vi "findLocation.vi"(10 "DAQmx \nPhysical Channel":tag="Dev2/ai0:31") -> (1 "Animals location":string)   [LabVIEW 2017]
panel:
  out "x/y 2":dbl
  out "max value":dbl
  out "sum":dbl
  out "max\nweights":dbl[](array[numeric])
  out "voltsPerGram":dbl[](array[numeric])
  out "zeroSignals":dbl[](array[numeric])
  out "load cell\nsignal":dbl[](array[numeric])
  in  "number of consecutive\nmeasurements":i32=10
  out "array w/ subset deleted":dbl[][](array[numeric])
  out "min \nweights":dbl[](array[numeric])
  out "appended array":dbl[][](array[numeric])
  out "x/y":dbl[](array[numeric])
  # "should be 10 for the rats"
  # "Channels to weigh"
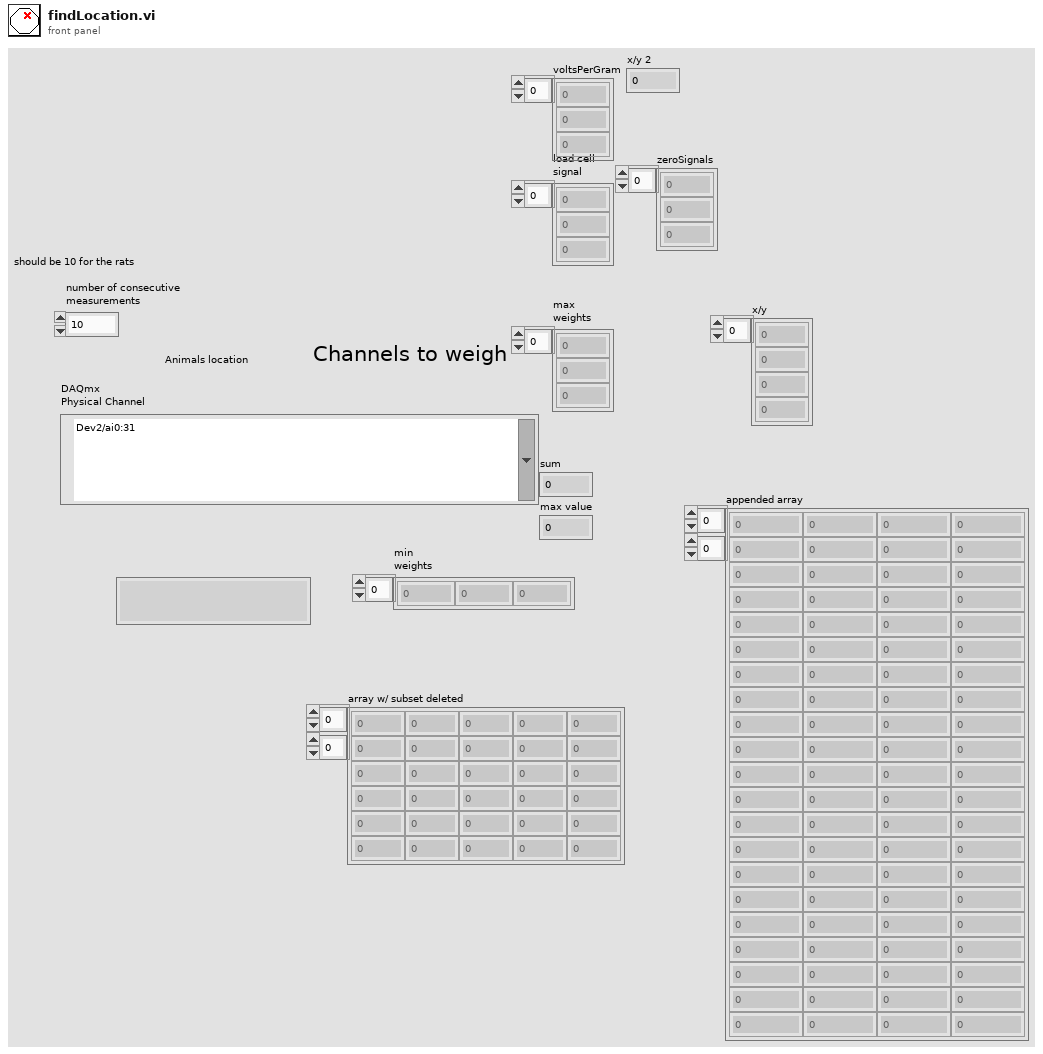
[diagram p1: front panel]
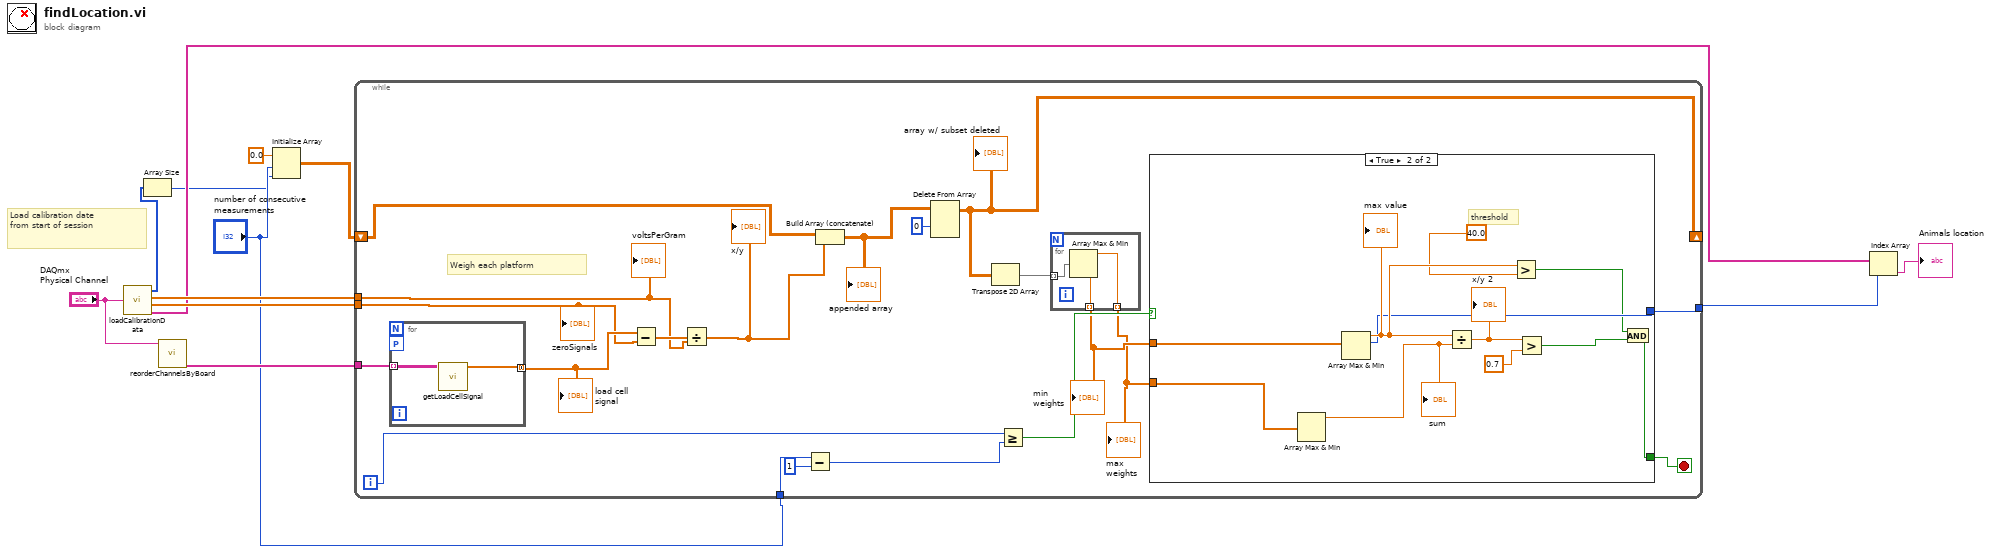
[diagram p0: block diagram]
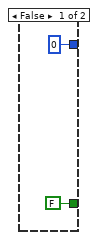
[diagram p2: hidden frame]
diagram:
  # "Load calibration date\nfrom start of session"
  n1 = call "loadCalibrationData.vi"("DAQmx \nPhysical Channel"="DAQmx \nPhysical Channel") -> ("channel names out"=w7:string[], "zeroSignals"=w12:dbl[], "voltsPerGram"=w11:dbl[], "index"=w4:i32[])  [unwired: 7 in]
  n2 = Array Size(array=w4) -> (size(s)=w1:i32)
  n3 = call "reorderChannelsByBoard.vi"("DAQmx \nPhysical Channel"="DAQmx \nPhysical Channel") -> ("Separated inputs\nas strings"=w9:string[])  [unwired: 8 in, 2 out]
  n4 = Initialize Array(0.0 ("element"), "number of consecutive\nmeasurements", w1) -> (w3:dbl[][])
  n5 = while {
    tunnel: w12 -> [w26]
    tunnel: w11 -> [w31]
    tunnel: w9 -> [w29]
    tunnel: [w28] -> w8
    shift-right: [w15] -> _
    shift-left: w3 -> [w24]
    tunnel: "number of consecutive\nmeasurements" -> [w17]
    i -> [w22]
    stop <- w27 stop-if-true
    # "Weigh each platform"
    n6 = for {
      workers-P: _ -> [_]
      tunnel: w29 -> [w50] mode=indexing
      tunnel: [w49] -> w30 mode=concatenating
      n7 = call "getLoadCellSignal.vi"("DAQmx Physical Channel"=w50) -> ("load cell\nsignal"=w49:dbl[])  [unwired: 10 in]
    }
    "load cell\nsignal" <- w30
    n8 = Subtract(x=w30, y=w26) -> (x-y=w32:dbl[])
    n9 = Divide(x=w32, y=w31) -> (x/y=w25:dbl[])
    "x/y" <- w25
    n10 = Subtract(x=w17, y=1) -> (x-y=w14:i32)
    n11 = Build Array (concatenate)(w24, w25) -> (w21:dbl[][])
    "appended array" <- w21
    n12 = Delete From Array(array=w21, index (row)=0) -> (array with subset deleted=w15:dbl[][])  [unwired: 2 in, 1 out]
    "array w/ subset deleted" <- w15
    n13 = Transpose 2D Array(2D array=w15) -> (transposed array=w18:dbl[][])
    n14 = Greater Or Equal?(x=w22, y=w14) -> (x >= y?=w23:bool)
    n15 = for {
      tunnel: w18 -> [w35] mode=indexing
      tunnel: [w34] -> w20 mode=indexing
      tunnel: [w33] -> w13 mode=indexing
      n16 = Array Max & Min(array=w35) -> (max value=w33:dbl, min value=w34:dbl)  [unwired: 2 out]
    }
    "min \nweights" <- w20
    "max\nweights" <- w13
    n17 = case shown="True" w23 {
      tunnel: [0 w42] -> w28
      tunnel: [FALSE w44] -> w27
      tunnel: w20 -> [_ w43]
      tunnel: w13 -> [_ w39]
      frame False {
      }
      frame True {
        # "threshold"
        n18 = Array Max & Min(array=w39) -> (max value=w38:dbl)  [unwired: 3 out]
        "sum" <- w38
        n19 = Array Max & Min(array=w43) -> (max value=w46:dbl, max index (indices)=w42:i32)  [unwired: 2 out]
        "max value" <- w46
        n20 = Divide(x=w46, y=w38) -> (x/y=w48:dbl)
        "x/y 2" <- w48
        n21 = Greater?(x=w46, y=40.0) -> (0:w40:bool)
        n22 = Greater?(x=w48, y=0.7) -> (0:w45:bool)
        n23 = And(x=w40, y=w45) -> (x .and. y?=w44:bool)
      }
    }
    "zeroSignals" <- w26
    "voltsPerGram" <- w31
  }
  n24 = Index Array(array=w7, index=w8) -> (element=→"Animals location":string)
